vi "Init Instrument.vi"(8 "error in":errorcluster, 11 "Source":string) -> (0 "error out":errorcluster, 2 "IInstrument out":refnum<class "IInstrument.lvclass">, 3 "Instrument Identifier":string)   [LabVIEW 2024, in "Instrument Manager.lvclass"]
uses:
  Instrument Manager.lvclass
  Instrument Manager.lvclass/Instrument Manager.ctl
  Instrument Factory/Instrument Factory.lvclass
  Config from JSON/Config from JSON.lvclass
  Config from XML/Config from XML.lvclass
  Interfaces/IConfigure/IStoreConfiguration.lvclass
  Interfaces/IInstrument/IInstrument.lvclass
  Interfaces/IConfigurable/IConfigurable.lvclass
  Interfaces/IConfigurationStrategy/IConfigurationStrategy.lvclass
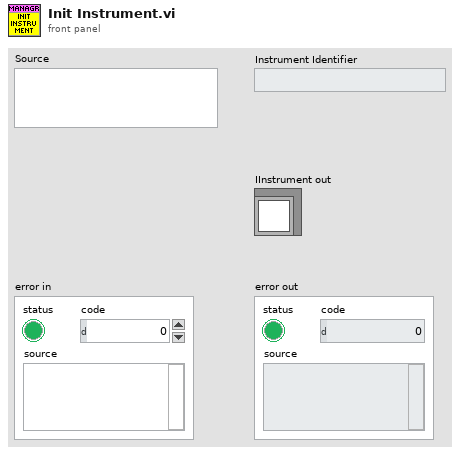
[diagram p1: front panel]
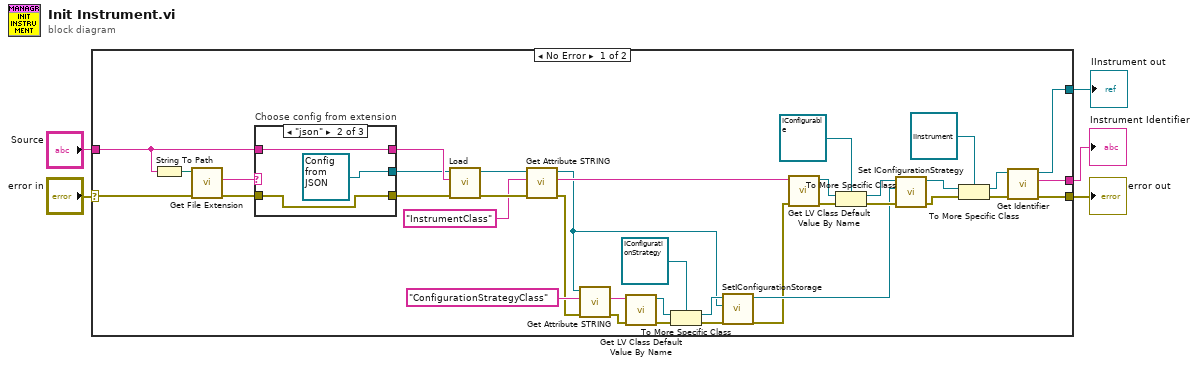
[diagram p0: block diagram]
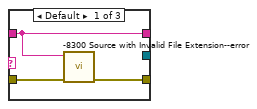
[diagram p2: hidden frame]
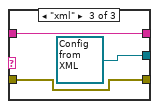
[diagram p3: hidden frame]
diagram:
  n1 = case shown="No Error" "error in" {
    selector: "error in" -> [w10 w50]
    tunnel: [w9 w50] -> w4
    tunnel: "Source" -> [w8 _]
    tunnel: [w7 _] -> w2
    tunnel: [w6 _] -> w1
    frame No Error {
      n2 = String To Path(string=w8) -> (path=w37:path)
      n3 = call <vilib>:"Get File Extension.vi"("error in (no error)"=w10, "file"=w37) -> ("error out"=w36:errorcluster, "lowercase file extension"=w40:string)  [unwired: 5 in, 3 out]
      n4 = case "Choose config from extension" shown="\"json\"" w40 {
        tunnel: w8 -> [w41 w46 w48]
        tunnel: [w41 w46 w48] -> w39
        tunnel: [_ refnum<class "Config from JSON.lvclass"> refnum ("Config from JSON.lvclass") refnum<class "Config from XML.lvclass"> refnum ("Config from XML.lvclass")] -> w38
        tunnel: w36 -> [w43 w44 w47]
        tunnel: [w42 w44 w47] -> w35
        frame Default {
          n5 = call "-8300 Source with Invalid File Extension--error.vi"("error in (no error)"=w43, "Source"=w41) -> ("error out"=w42:errorcluster)  [unwired: 9 in]
        }
        frame "json" {
        }
        frame "xml" {
        }
      }
      n6 = call-dynamic "Load.vi"("error in"=w35, "Source"=w39, "IStoreConfiguration in"=w38) -> ("error out"=w33:errorcluster, "IStoreConfiguration out"=w34:refnum<class "IStoreConfiguration.lvclass">)  [unwired: 7 in]
      n7 = call-dynamic "Get Attribute STRING.vi"("error in"=w33, "Attribute"="InstrumentClass", "IStoreConfiguration in"=w34) -> ("error out"=w16:errorcluster, "Value"=w31:string, "IStoreConfiguration out"=w18:refnum<class "IStoreConfiguration.lvclass">)  [unwired: 6 in]
      n8 = call-dynamic "Get Attribute STRING.vi"("error in"=w16, "Attribute"="ConfigurationStrategyClass", "IStoreConfiguration in"=w18) -> ("error out"=w23:errorcluster, "Value"=w24:string)  [unwired: 6 in, 1 out]
      n9 = call <vilib>:"Get LV Class Default Value By Name.vi"("error in (no error)"=w23, "class name"=w24) -> ("error out"=w22:errorcluster, "object"=w21:refnum<class>)  [unwired: 8 in]
      n10 = To More Specific Class(target class=refnum<class "IConfigurationStrategy.lvclass"> refnum ("IConfigurationStrategy.lvclass"), reference=w21, error in=w22) -> (specific class reference=w19:refnum<class "IConfigurationStrategy.lvclass">, error out=w15:errorcluster)
      n11 = call-dynamic "SetIConfigurationStorage.vi"("IStoreConfiguration"=w18, "IConfigurationStrategy in"=w19) -> ("IConfigurationStrategy out"=w17:refnum<class "IConfigurationStrategy.lvclass">)  [unwired: 9 in]
      n12 = call <vilib>:"Get LV Class Default Value By Name.vi"("error in (no error)"=w15, "class name"=w31) -> ("error out"=w29:errorcluster, "object"=w30:refnum<class>)  [unwired: 8 in]
      n13 = To More Specific Class(target class=refnum<class "IConfigurable.lvclass"> refnum ("IConfigurable.lvclass"), reference=w30, error in=w29) -> (specific class reference=w28:refnum<class "IConfigurable.lvclass">, error out=w26:errorcluster)
      n14 = call-dynamic "Set IConfigurationStrategy.vi"("IConfigurationStrategy"=w17, "IConfigurable in"=w28) -> ("IConfigurable out"=w27:refnum<class "IConfigurable.lvclass">)  [unwired: 9 in]
      n15 = To More Specific Class(target class=refnum<class "IInstrument.lvclass"> refnum ("IInstrument.lvclass"), reference=w27, error in=w26) -> (specific class reference=w11:refnum<class "IInstrument.lvclass">, error out=w14:errorcluster)
      n16 = call-dynamic "Get Identifier.vi"("error in"=w14, "IInstrument in"=w11) -> ("error out"=w9:errorcluster, "Identifier"=w6:string, "IInstrument out"=w7:refnum<class "IInstrument.lvclass">)  [unwired: 7 in]
    }
    frame Error {
    }
  }
  "error out" <- w4
  "IInstrument out" <- w2
  "Instrument Identifier" <- w1
